vi "ScanDirection.vi"() -> ()   [LabVIEW 2011]
panel:
  in  "ScanDirection":enum32{"X-Y", "X-Z", "Y-Z", "Focus"}(radio)
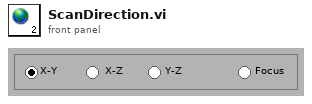
[diagram p1: front panel]
diagram:
